vi "Image Acquire.vi"(0 "Image Dir Path":path caption="Image Path", 3 "Next":bool, 7 "error in":errorcluster) -> (20 "Image Out":T1(plugin-control), 22 "ImageIndex":i32, 27 "error out":errorcluster)   [LabVIEW 2015]
doc: "Creates, and edits acquisitions using the NI Vision Acquisition Express VI.\n\nThe NI Vision Acquisition Wizard is launched by placing the Express VI on the block diagram. Select an acquisition source and configure an acquisition using NI-IMAQ, NI-IMAQdx, or simulate an acquisition by reading an AVI or image files from a folder. After an acquisition is configured, select controls and indicators to be able to programmatically set in LabVIEW. Double-click the Vision Acquisition Express VI to edit the acquisition.\n\nNote: Any images created by the Express VI need to be disposed after use. Use the IMAQ Dispose.vi to cleanup the images output by the Express VI when they are no longer needed."
uses:
  Controls/BELKIN RT State.ctl
  Stream/LP Globals.vi
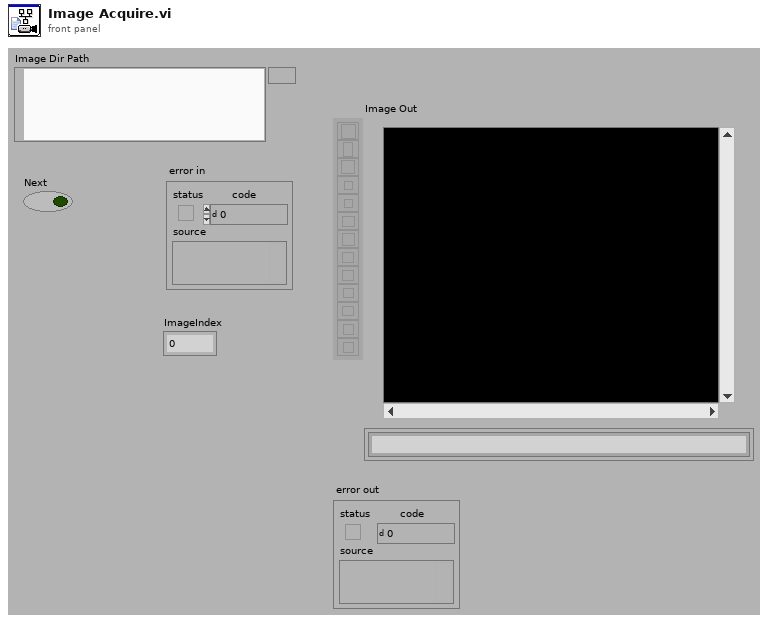
[diagram p1: front panel]
types:
  T1 = typedef "IMAQ Image.ctl" = refnum<image>
  T2 = typedef "BELKIN RT State.ctl" = enum16{"Initialize", "BIT", "Warm Up", "Eye Location", "Find Limbus", "Eye Track", "Fire", "Treatment Complete", "Shut Down", "Error"}
  T3 = typedef "Image Type" = u32
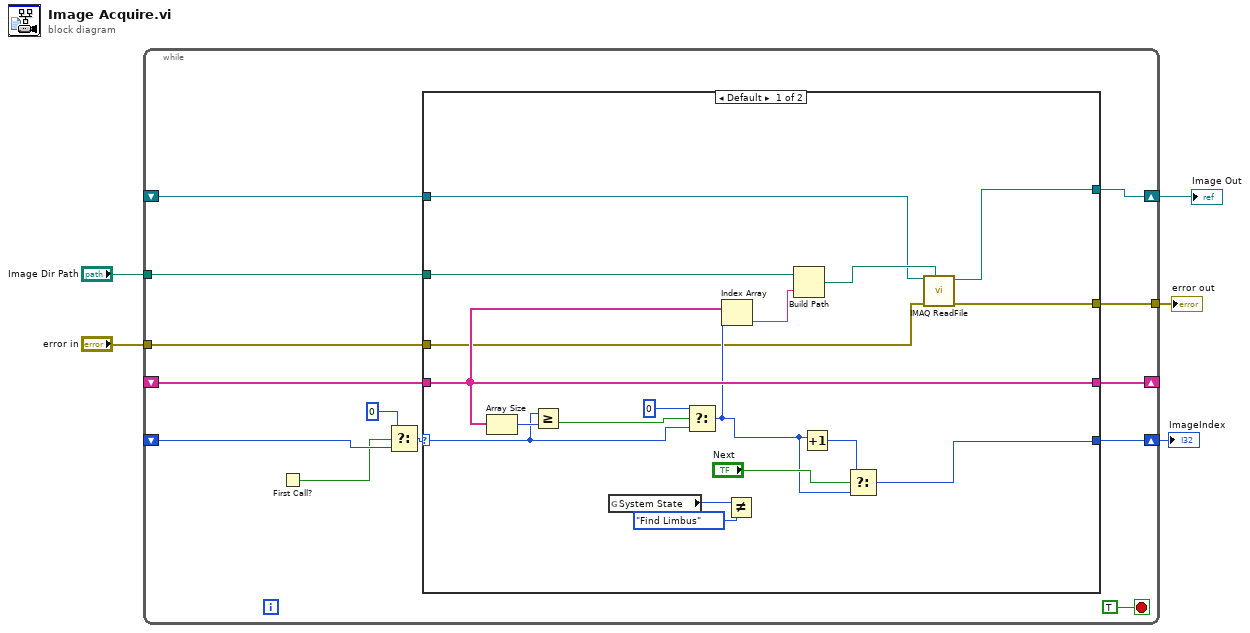
[diagram p0: block diagram]
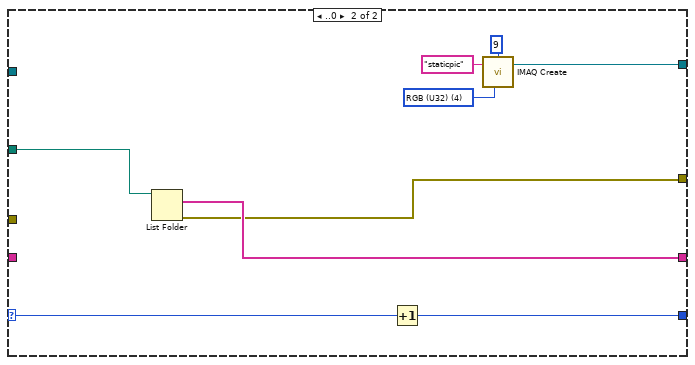
[diagram p2: hidden frame]
diagram:
  n1 = while {
    tunnel: [w18] -> w5
    shift-right: [w13] -> w2
    shift-left: _ -> [w12]
    shift-right: [w17] -> _
    shift-left: _ -> [w11]
    tunnel: "Image Dir Path" -> [w16]
    tunnel: "error in" -> [w10]
    shift-right: [w7] -> w1
    shift-left: _ -> [w6]
    stop <- TRUE stop-if-true
    n2 = First Call?() -> (First Call?: T/F=w8:bool)
    n3 = Select(t=0, s=w8, f=w12) -> (s? t:f=w14:i32)
    n4 = case shown="Default" w14 {
      selector: w14 -> [w35 w43]
      tunnel: [w33 w41] -> w18
      tunnel: [w29 w45] -> w17
      tunnel: w16 -> [w32 w44]
      tunnel: [w23 w42] -> w13
      tunnel: w11 -> [w29 _]
      tunnel: w10 -> [w22 _]
      tunnel: [w20 w37] -> w7
      tunnel: w6 -> [w21 _]
      frame Default {
        n5 = Array Size(array=w29) -> (size(s)=w36:i32)
        n6 = Greater Or Equal?(x=w35, y=w36) -> (x >= y?=w19:bool)
        n7 = global read "LP Globals.vi" "System State"() -> (w28:T2)
        n8 = Select(t=0, s=w19, f=w35) -> (s? t:f=w24:i32)
        n9 = Index Array(array=w29, index=w24) -> (element=w31:string)
        n10 = Not Equal?(x=w28, y=BELKIN_RT_State."Find Limbus") -> ()  [unwired: 1 out]
        n11 = Build Path(base path=w32, name or relative path=w31) -> (appended path=w30:path)
        n12 = Increment(x=w24) -> (x+1=w25:i32)
        n13 = Select(t=w25, s="Next", f=w24) -> (s? t:f=w23:i32)
        n14 = call "IMAQ ReadFile"("File Path"=w30, "error in (no error)"=w22, "Image"=w21) -> ("error out"=w33:errorcluster, "Image Out"=w20:T1)  [unwired: 2 in, 5 out]
      }
      frame ..0 {
        w39 = T3 4 items=["Grayscale (U8)", "Grayscale (I16)", "Grayscale (SGL)", "Complex (CSG)", "RGB (U32)", "HSL (U32)", "RGB (U64)", "Grayscale (U16)"] ("Image Type")
        n15 = List Folder(path=w44) -> (filenames=w45:string[], error out=w41:errorcluster)  [unwired: 3 in, 2 out]
        n16 = Increment(x=w43) -> (x+1=w42:i32)
        n17 = call "IMAQ Create"("Border Size"=9, "Image Name"="staticpic", "Image Type"=w39) -> ("New Image"=w37:T1)  [unwired: 1 in, 2 out]
      }
    }
  }
  "error out" <- w5
  "ImageIndex" <- w2
  "Image Out" <- w1
